vi "Build File Name.vi"(8 "error in (no error)":errorcluster, 11 "Text File Sink in":refnum<class "Text File Sink.lvclass">) -> (0 "error out":errorcluster, 3 "Text File Sink out":refnum<class "Text File Sink.lvclass">)   [LabVIEW 2020, in "MVA Framework.lvlib" / "Text File Sink.lvclass"]
uses:
  Text File Sink.lvclass
  Text File Sink.lvclass/Text File Sink.ctl
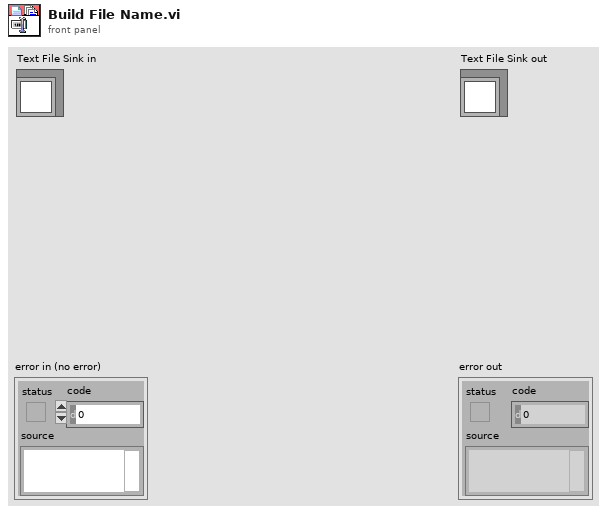
[diagram p1: front panel]
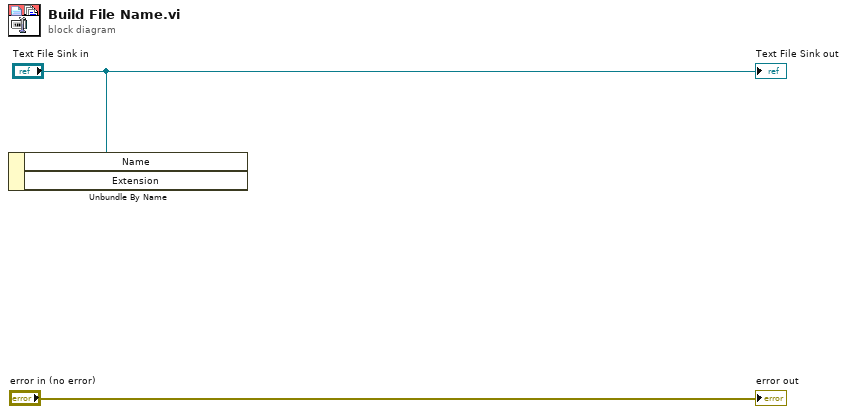
[diagram p0: block diagram]
diagram:
  n1 = Unbundle By Name("Text File Sink in") -> ()  [unwired: 2 out]
  "error out" <- "error in (no error)"
  "Text File Sink out" <- "Text File Sink in"
